vi "Keysight_ATI40.vi"() -> ()   [LabVIEW 2023]
uses:
  <vilib>/Analysis/baseanly.llb/A x Vector.vi
  <vilib>/Utility/file.llb/Write To Spreadsheet File (DBL).vi
  <instrlib>/Agilent 34970/Agilent 34970.lvlib
  <vilib>/Analysis/NI_AALBase.lvlib
panel:
  in  "Transform":T1
  in  "Torque Units":string="N-m"
  in  "Force Units":string="N"
  in  "Calibration File":path=path "C:/Users/d066566/OneDrive - Politecnico di Torino/PhD/PhD/Test files/Denver/FT17838/FT17838.cal"
  out "Raw Voltages":dbl[](array[numeric]) format="%.2f"
  out "error out":errorcluster
  in  "Save":bool
  in  "Data File":path=path "C:/Users/d066566/Desktop/asdf3.csv"
  in  "Data format and type":string="%.6f"
  in  "stop":bool
  in  "VISA resource name":refnum<visa-resource-name>="GPIB0::9::INSTR"
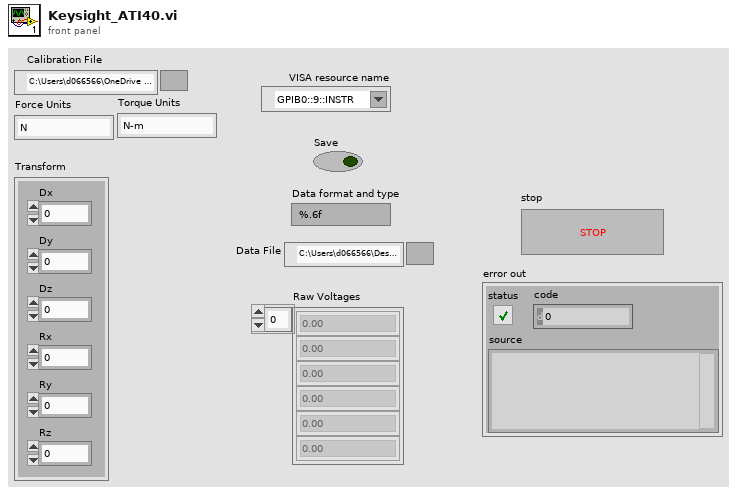
[diagram p1: front panel]
types:
  T1 = cluster{"Dx":dbl, "Dy":dbl, "Dz":dbl, "Rx":dbl, "Ry":dbl, "Rz":dbl}
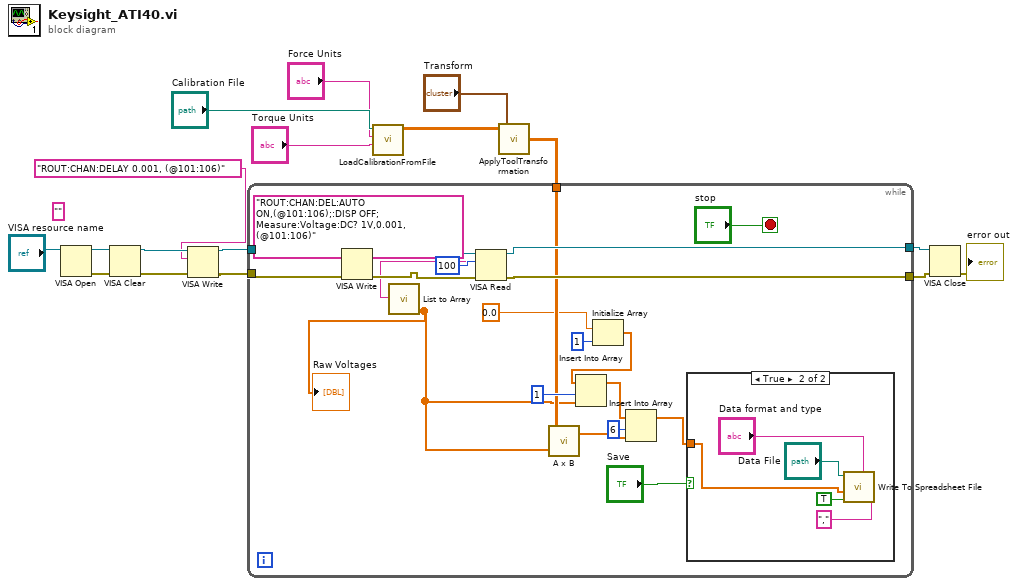
[diagram p0: block diagram]
diagram:
  (unwired) ""
  n1 = VISA Open(VISA resource name="VISA resource name") -> (VISA resource name=w16:refnum<visa-resource-name>, error out=w15:errorcluster)  [unwired: 4 in]
  n2 = VISA Clear(VISA resource name=w16, error in (no error)=w15) -> (VISA resource name out=w3:refnum<visa-resource-name>, error out=w2:errorcluster)
  n3 = VISA Write(VISA resource name=w3, write buffer="ROUT:CHAN:DELAY 0.001, (@101:106)", error in (no error)=w2) -> (VISA resource name out=w5:refnum<visa-resource-name>, error out=w4:errorcluster)  [unwired: 1 out]
  n4 = call <instrlib>:"LoadCalibrationFromFile.vi"("User Torque Units"="Torque Units", "User Force Units"="Force Units", "Cal File Path"="Calibration File") -> ("Calibration Matrix"=w8:dbl[][])  [unwired: 1 in, 3 out]
  n5 = call <instrlib>:"ApplyToolTransformation.vi"("Transform"="Transform", "Calibration Matrix"=w8) -> ("Transformed Calibration Matrix"=w6:dbl[][])
  n6 = while {
    tunnel: [w36] -> w14
    tunnel: [w35] -> w13
    tunnel: w4 -> [w28]
    tunnel: w5 -> [w27]
    tunnel: w6 -> [w26]
    stop <- "stop" stop-if-true
    n7 = VISA Write(VISA resource name=w27, write buffer="ROUT:CHAN:DEL:AUTO ON,(@101:106);:DISP OFF; Measure:Voltage:DC? 1V,0.001,  (@101:106)", error in (no error)=w28) -> (VISA resource name out=w32:refnum<visa-resource-name>, error out=w33:errorcluster)  [unwired: 1 out]
    n8 = VISA Read(VISA resource name=w32, byte count=u32 100, error in (no error)=w33) -> (VISA resource name out=w35:refnum<visa-resource-name>, read buffer=w31:string, error out=w36:errorcluster)  [unwired: 1 out]
    n9 = call <instrlib>:"List to Array.vi"("List (empty)"=w31) -> ("Output Number Array"=w21:dbl[])  [unwired: 9 in, 1 out]
    "Raw Voltages" <- w21
    n10 = call-poly <vilib>:"A x B.vi"("Vector"=w21, "A"=w26) -> ("A x Vector"=w24:dbl[])  [unwired: 1 out]
    n11 = Initialize Array(0.0 ("element"), 1 ("dimension size")) -> (w22:dbl[])
    n12 = Insert Into Array(array=w22, index=1, new element=w21) -> (w20:dbl[])
    n13 = Insert Into Array(array=w20, index=6, new element=w24) -> (w23:dbl[])
    n14 = case shown="True" "Save" {
      tunnel: w23 -> [_ w39]
      frame False {
      }
      frame True {
        n15 = call-poly <vilib>:"Write To Spreadsheet File.vi"("delimiter (\\t)"=",", "format (%.3f)"="Data format and type", "append to file? (new file:F)"=TRUE, "1D data"=w39, "file path (dialog if empty)"="Data File") -> ()  [unwired: 3 in, 1 out]
      }
    }
  }
  n16 = VISA Close(VISA resource name=w13, error in (no error)=w14) -> (error out=→"error out":errorcluster)
